vi "WLAN Configure Standard.vi"(0 "Instrument Handle In":refnum<k21>, 1 "Selector String":string, 5 "WLAN Standard Configuration":T1={"Standard"=0, "Channel Bandwidth (Hz)"=20000000.0} {"Channel Bandwidth (Hz)" items=["5M"=5000000.0, "10M"=10000000.0, "20M"=20000000.0, "40M"=40000000.0, "80M"=80000000.0, "160M"=160000000.0]; "Standard" items=["802.11a/g", "802.11b", "802.11j", "802.11p", "802.11n", "802.11ac", "802.11ax"]}, 11 "error in (no error)":errorcluster) -> (4 "Instrument Handle Out":refnum<k21>, 15 "error out":errorcluster)   [LabVIEW 2016, in "RFmxWLAN.lvlib"]
doc: "Configures common settings related to the WLAN standard of the measured signal."
uses:
  RFmxWLAN.lvlib
  Typedefs/WLAN Standard Configuration.ctl
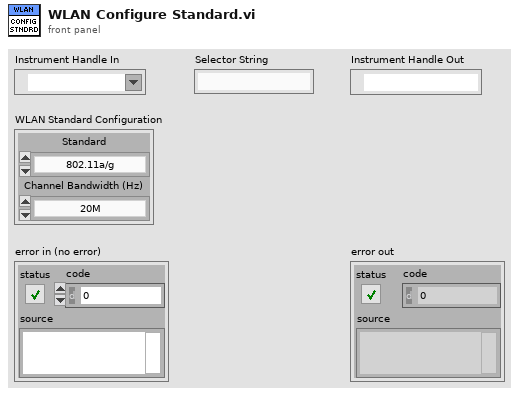
[diagram p1: front panel]
types:
  T1 = typedef "RFmxWLAN.lvlib/WLAN Standard Configuration.ctl" = cluster{"Standard":i32, "Channel Bandwidth (Hz)":dbl}
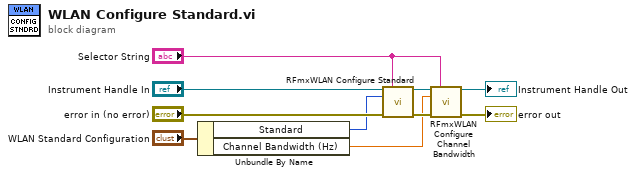
[diagram p0: block diagram]
diagram:
  n1 = Unbundle By Name("WLAN Standard Configuration") -> ("Standard"=w2:i32, "Channel Bandwidth (Hz)"=w1:dbl)
  n2 = call <vilib>:"RFmxWLAN Configure Standard.vi"("Instrument Handle In"="Instrument Handle In", "Selector String"="Selector String", "Standard"=w2, "error in (no error)"="error in (no error)") -> ("Instrument Handle Out"=w5:refnum<k21>, "error out"=w7:errorcluster)  [unwired: 10 in]
  n3 = call <vilib>:"RFmxWLAN Configure Channel Bandwidth.vi"("Instrument Handle In"=w5, "Selector String"="Selector String", "Channel Bandwidth (Hz)"=w1, "error in (no error)"=w7) -> ("Instrument Handle Out"=→"Instrument Handle Out":refnum<k21>, "error out"=→"error out":errorcluster)  [unwired: 10 in]
